vi "8bit-to-binary.vi"() -> ()   [LabVIEW 2013]
panel:
  out "Boolean array":bool[](array[boolean])
  in  "number":i8
  out "element":bool
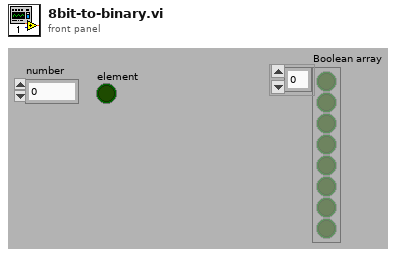
[diagram p1: front panel]
types:
  T1 = cluster{"Boolean array[0]":bool, "Boolean array[1]":bool, "Boolean array[2]":bool, "Boolean array[3]":bool, "Boolean array[4]":bool, "Boolean array[5]":bool, "Boolean array[6]":bool, "Boolean array[7]":bool}
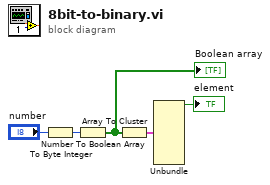
[diagram p0: block diagram]
diagram:
  n1 = To Byte Integer(number="number") -> (8bit integer=w3:i8)
  n2 = Number To Boolean Array(number=w3) -> (Boolean array=w1:bool[])
  "Boolean array" <- w1
  n3 = Array To Cluster(array=w1) -> (cluster=w5:T1)
  n4 = Unbundle(w5) -> ("Boolean array[0]"=→"element":bool)  [unwired: 7 out]
